vi "Write Inherited timeout.vi"(8 "error in (no error)":errorcluster, 10 "Inherited timeout":i32=-1, 11 "BaseMessage in":refnum<class "BaseMessage.lvclass">) -> (0 "error out":errorcluster, 3 "BaseMessage out":refnum<class "BaseMessage.lvclass">)   [LabVIEW 2013, in "BaseMessage.lvclass"]
doc: "Timeout (inherited from the reader) that will be used if the message has no other specified timeout"
uses:
  BaseMessage.lvclass
  BaseMessage.lvclass/BaseMessage.ctl
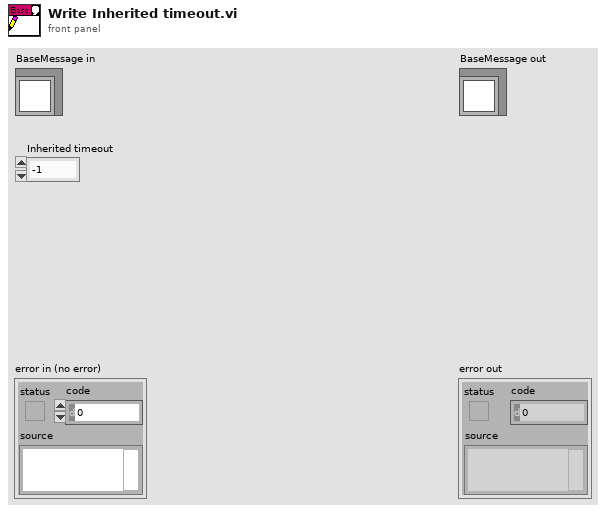
[diagram p1: front panel]
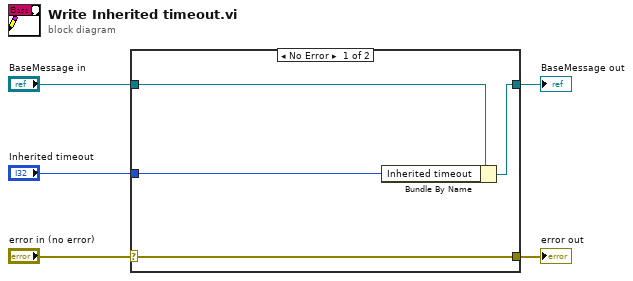
[diagram p0: block diagram]
diagram:
  n1 = case shown="No Error" "error in (no error)" {
    selector: "error in (no error)" -> [w9 w10]
    tunnel: [w9 w10] -> w4
    tunnel: [w7 w11] -> w2
    tunnel: "BaseMessage in" -> [w8 w11]
    tunnel: "Inherited timeout" -> [w6 _]
    frame No Error {
      n2 = Bundle By Name(cluster=w8, "Inherited timeout"=w6) -> (w7:refnum<class "BaseMessage.lvclass">)
    }
    frame Error {
    }
  }
  "error out" <- w4
  "BaseMessage out" <- w2
